vi "FGV_SQL_part_ID_buffer.vi"(4 "recordset_in":variant[][](array[variant]), 6 "connection reference":T2, 7 "options":T3, 8 "error_in":errorcluster, 9 "station":T1, 11 "PART_SERIAL":string) -> (0 "error_out":errorcluster, 2 "Part exists?":bool, 3 "ID_out":string)   [LabVIEW 2020]
uses:
  FGV_SQL_part_ID_buffer.ctl
  <vilib>/addons/database/Connection.llb/Conn ObjectReference.ctl
  STATION/station.ctl
  SQL_part_ID_buffer_all_info.ctl
  <vilib>/addons/database/NI_Database_API.lvlib
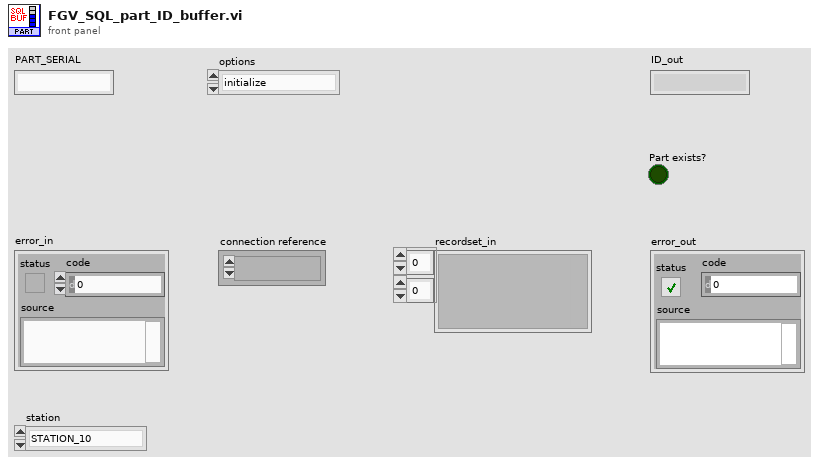
[diagram p1: front panel]
types:
  T1 = typedef "station.ctl" = enum16{"STATION_10", "STATION_20", "STATION_30", "STATION_40", "STATION_50", "STATION_60", "STATION_70", "STATION_80", "STATION_90", "STATION_100", "STATION_110", "STATION_120", "STATION_165", "MAIN"}
  T2 = typedef "NI_Database_API.lvlib/Conn ObjectReference.ctl" = refnum<k1>
  T3 = typedef "FGV_SQL_part_ID_buffer.ctl" = enum16{"initialize", "buffer_serial_ID", "get_ID_for_name"}
  T4 = typedef "SQL_part_ID_buffer_all_info.ctl" = cluster{"PART_SERIAL_and_ID":string[][], "PART_SERIAL_and_ID_buffer_pos":i32, "PART_SERIAL_and_ID_buffer_max_size":i32}
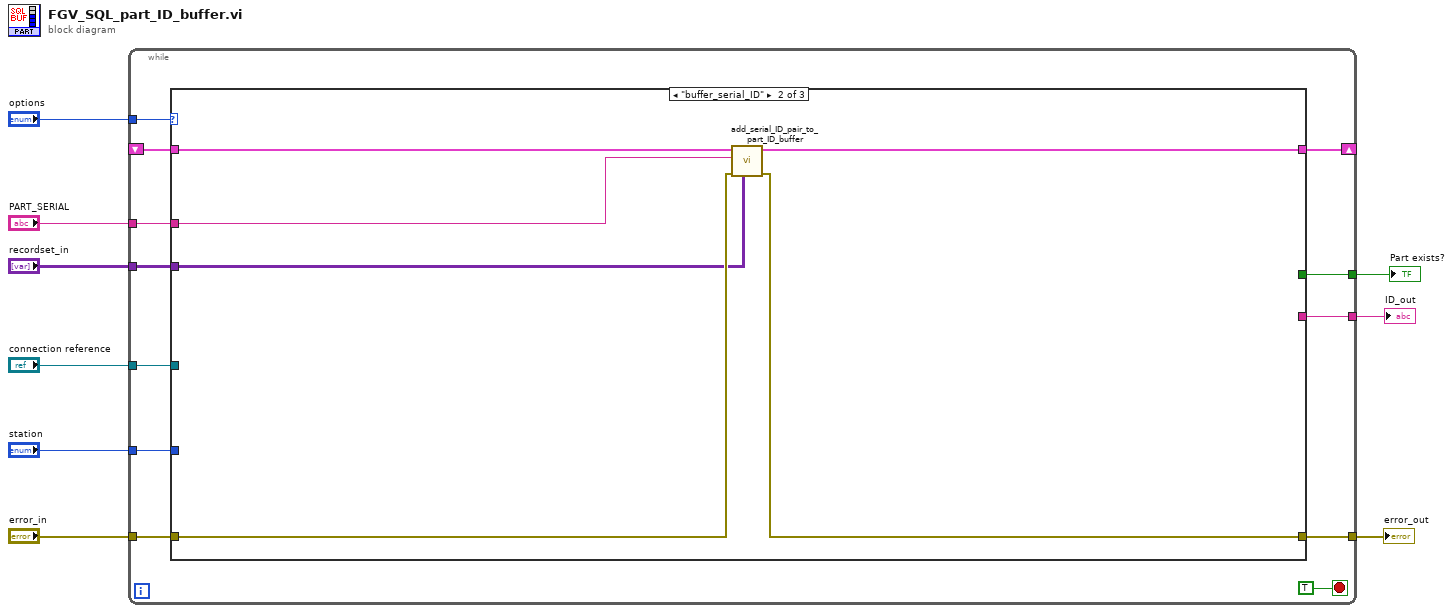
[diagram p0: block diagram]
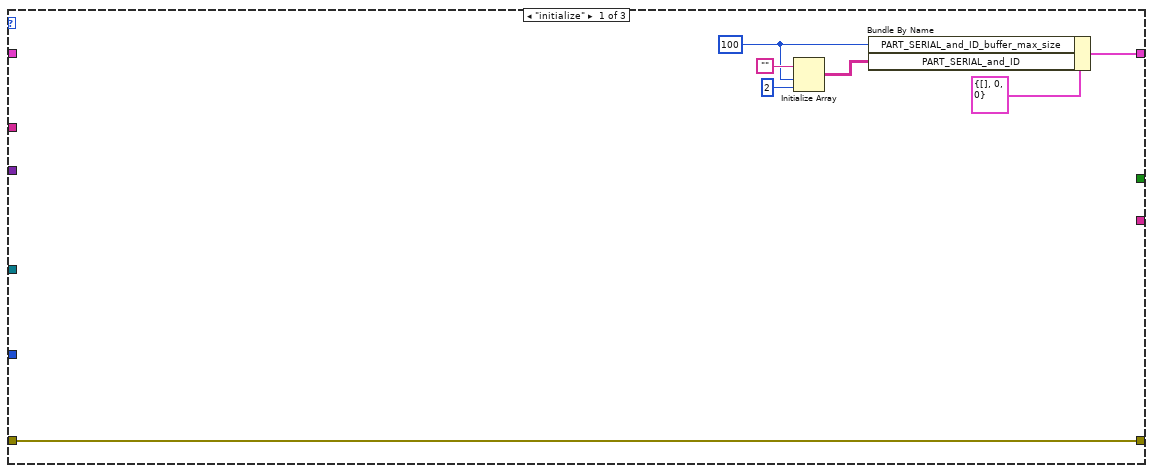
[diagram p2: hidden frame]
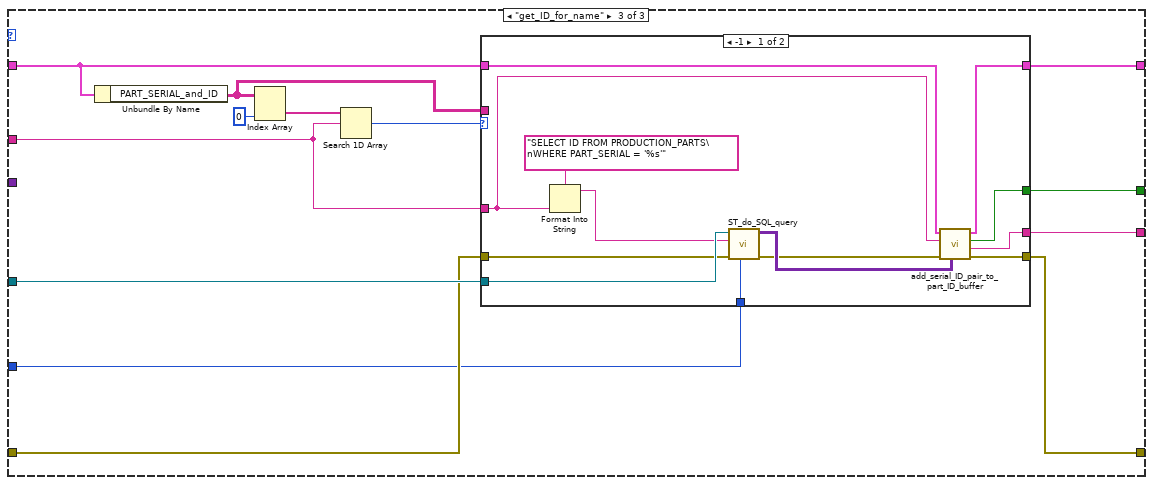
[diagram p3: hidden frame]
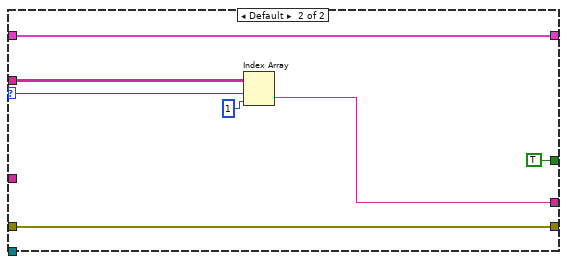
[diagram p4: hidden frame]
diagram:
  n1 = while {
    tunnel: "options" -> [w20]
    tunnel: [w19] -> w9
    tunnel: "error_in" -> [w18]
    shift-right: [w17] -> _
    shift-left: _ -> [w16]
    tunnel: "connection reference" -> [w13]
    tunnel: "PART_SERIAL" -> [w14]
    tunnel: "recordset_in" -> [w15]
    tunnel: [w12] -> w4
    tunnel: [w11] -> w2
    tunnel: "station" -> [w10]
    stop <- TRUE stop-if-true
    n2 = case shown="\"buffer_serial_ID\"" w20 {
      tunnel: [w28 w30 w39] -> w19
      tunnel: w18 -> [w28 w31 w40]
      tunnel: [w23 w32 w37] -> w17
      tunnel: w16 -> [_ w33 w38]
      tunnel: w15 -> [_ w29 _]
      tunnel: w14 -> [_ w34 w41]
      tunnel: w13 -> [_ _ w42]
      tunnel: [_ _ w43] -> w12
      tunnel: [_ _ w36] -> w11
      tunnel: w10 -> [_ _ w35]
      frame "initialize" {
        w22 = 100 ("dimension size")
        n3 = Initialize Array("", w22, 2 ("dimension size")) -> (w26:string[][])
        n4 = Bundle By Name(cluster=T4 {"PART_SERIAL_and_ID"=[], "PART_SERIAL_and_ID_buffer_pos"=0, "PART_SERIAL_and_ID_buffer_max_size"=0} ("SQL_EDIT_all_info"), "PART_SERIAL_and_ID_buffer_max_size"=w22, "PART_SERIAL_and_ID"=w26) -> (w23:T4)
      }
      frame "buffer_serial_ID" {
        n5 = call "add_serial_ID_pair_to_part_ID_buffer.vi"("recordset_in"=w29, "error_in"=w31, "PART_SERIAL"=w34, "SQL_part_ID_buffer_all_info_in"=w33) -> ("error_out"=w30:errorcluster, "SQL_part_ID_buffer_all_info_out"=w32:T4)  [unwired: 4 in, 2 out]
      }
      frame "get_ID_for_name" {
        n6 = Unbundle By Name(w38) -> ("PART_SERIAL_and_ID"=w44:string[][])
        n7 = Index Array(array=w44, index (col)=0 ("disabled index (col)")) -> (element=w46:string[])  [unwired: 1 in]
        n8 = Search 1D Array(1D array=w46, element=w41) -> (index of element=w45:i32)  [unwired: 1 in]
        n9 = case shown="-1" w45 {
          selector: w45 -> [_ w67]
          tunnel: w44 -> [_ w66]
          tunnel: [w55 w64] -> w43
          tunnel: w42 -> [w54 _]
          tunnel: w41 -> [w56 _]
          tunnel: w40 -> [w51 w63]
          tunnel: [w59 w63] -> w39
          tunnel: w38 -> [w58 w62]
          tunnel: [w57 w62] -> w37
          tunnel: [w53 TRUE ("Part exists?")] -> w36
          tunnel: w35 -> [w49 _]
          frame -1 {
            n10 = Format Into String(format string="SELECT ID FROM PRODUCTION_PARTS\nWHERE PART_SERIAL = '%s'", w56) -> (resulting string=w50:string)  [unwired: 2 in, 1 out]
            n11 = call "ST_do_SQL_query.vi"("station"=w49, "error_in"=w51, "SQL_query"=w50, "SQL_connection_reference"=w54) -> ("error_out"=w48:errorcluster, "recordset_out"=w52:variant[][])  [unwired: 6 in]
            n12 = call "add_serial_ID_pair_to_part_ID_buffer.vi"("recordset_in"=w52, "error_in"=w48, "PART_SERIAL"=w56, "SQL_part_ID_buffer_all_info_in"=w58) -> ("error_out"=w59:errorcluster, "PART_ID_out"=w55:string, "Part exists?"=w53:bool, "SQL_part_ID_buffer_all_info_out"=w57:T4)  [unwired: 4 in]
          }
          frame Default {
            n13 = Index Array(array=w66, index (row)=w67, index (col)=1 ("disabled index (col)")) -> (element=w64:string)
          }
        }
      }
    }
  }
  "error_out" <- w9
  "ID_out" <- w4
  "Part exists?" <- w2
